vi "DisplayErrorsToUser.vi"() -> ()   [LabVIEW 2011]
panel:
  out "Current Number of Errors:\nOnly Returns the Last 100":i32
  in  "Cancel Button":bool
  out "Error source":string[](array[string])
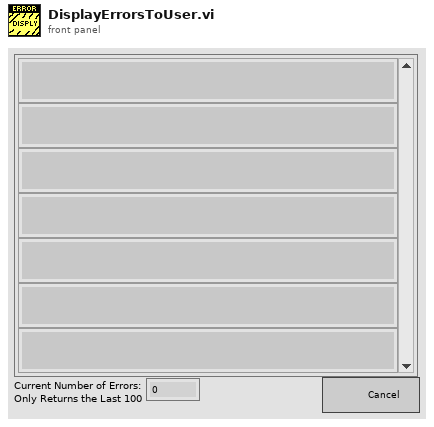
[diagram p1: front panel]
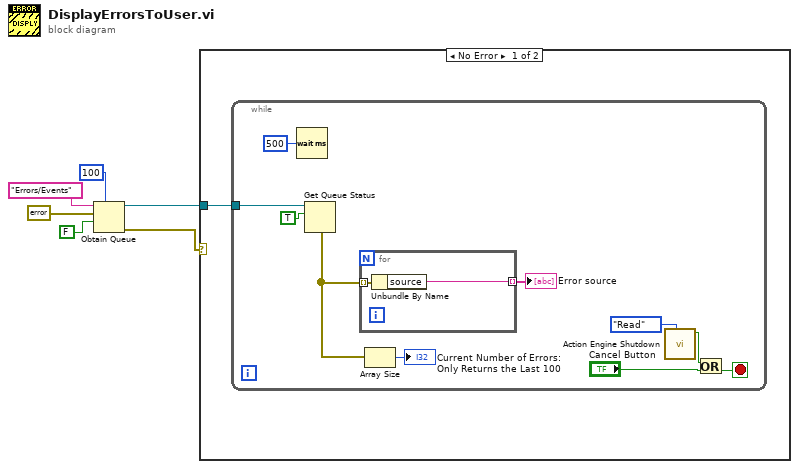
[diagram p0: block diagram]
diagram:
  n1 = Obtain Queue(max queue size (-1, unlimited)=100, name (unnamed)="Errors/Events", element data type=errorcluster {"status"=FALSE, "code"=0, "source"=""} ("error constant"), create if not found? (T)=FALSE) -> (queue out=w4:refnum<queue>, error out=w1:errorcluster)  [unwired: 1 in, 1 out]
  n2 = case shown="No Error" w1 {
    tunnel: w4 -> [w7 _]
    frame No Error {
      n3 = while {
        tunnel: w7 -> [w17]
        stop <- w9 stop-if-true
        n4 = Wait (ms)(milliseconds to wait=u32 500) -> ()  [unwired: 1 out]
        n5 = Get Queue Status(queue=w17, return elements? (F)=TRUE) -> (elements=w12:errorcluster[])  [unwired: 1 in, 7 out]
        n6 = for {
          tunnel: w12 -> [w19] mode=indexing
          tunnel: [w18] -> w14 mode=indexing
          n7 = Unbundle By Name(w19) -> ("source"=w18:string)
        }
        "Error source" <- w14
        n8 = Array Size(array=w12) -> (size(s)=→"Current Number of Errors:\nOnly Returns the Last 100":i32)
        n9 = call "Action Engine Shutdown.vi"("Shutdown"=enum16{"Write", "Read"}."Read") -> ("Shutdown"=w8:bool)  [unwired: 9 in, 1 out]
        n10 = Or(x=w8, y="Cancel Button") -> (x .or. y?=w9:bool)
      }
    }
    frame Error {
    }
  }
